vi "Save File Save Current.vi"(8 "Timer Seconds":dbl, 9 "Voltage":dbl, 10 "File Locations":T1, 11 "Current":dbl) -> (3 "Saving":bool)   [LabVIEW 2018, in "Save File.lvlib"]
uses:
  Save File.lvlib
  File Setup (Public)/Type Definition/Save File DOE File Path Control.ctl
  File Setup (Public)/Type Definition/Save File DOE Data Save Filepaths.ctl
  <vilib>/Utility/file.llb/Write To Spreadsheet File (string).vi
  <vilib>/Utility/file.llb/Write Delimited Spreadsheet (string).vi
  File Setup.lvlib
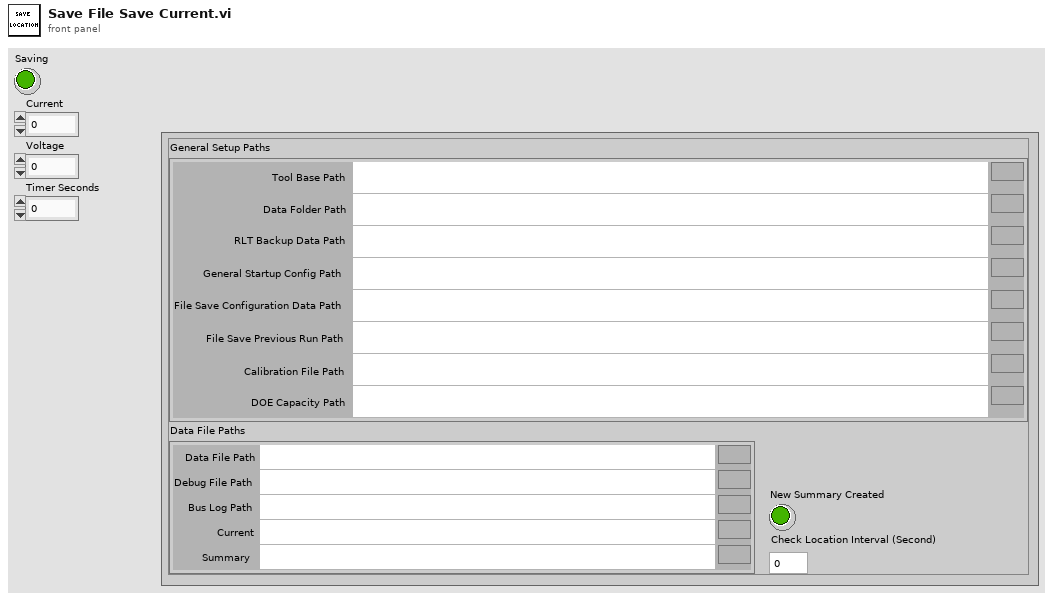
[diagram p1: front panel]
types:
  T1 = typedef "File Setup.lvlib/Save File DOE File Path Control.ctl" = cluster{"General Setup Paths":cluster{"Calibration File Path":path, "DOE Capacity Path":path, "Data Folder Path":path, "RLT Backup Data Path":path, "Tool Base Path":path, "General Startup Config Path":path, "File Save Previous Run Path":path, "File Save Configuration Data Path":path}, "Data File Paths":T2, "New Summary Created":bool, "Check Location Interval (Second)":i32}
  T2 = typedef "File Setup.lvlib/Save File DOE Data Save Filepaths.ctl" = cluster{"Data File Path":path, "Debug File Path":path, "Bus Log Path":path, "Current":path, "Summary":path}
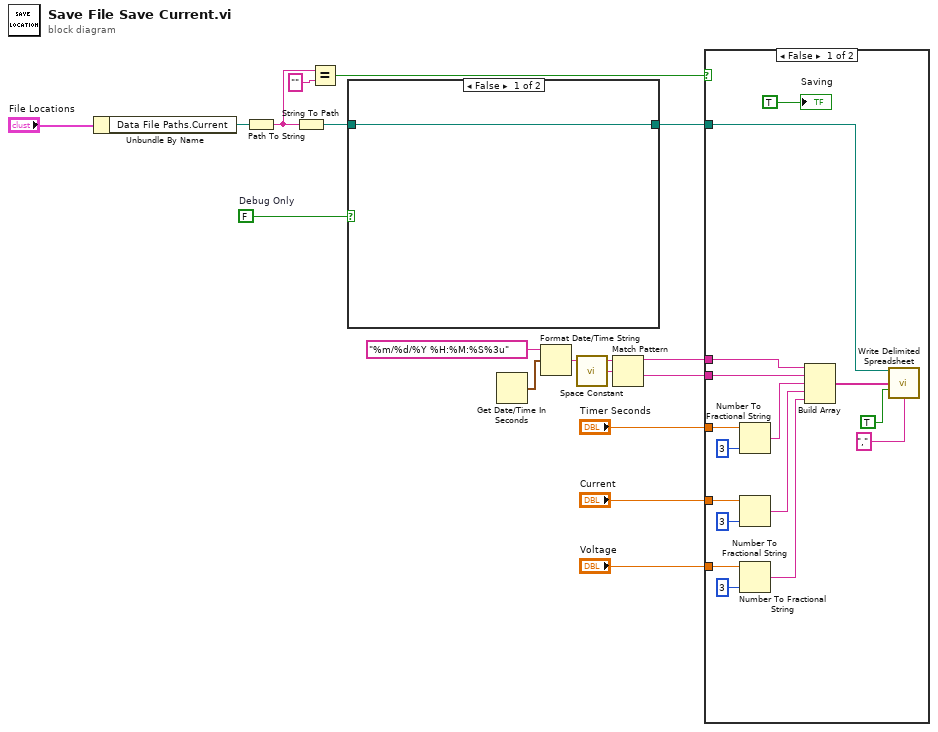
[diagram p0: block diagram]
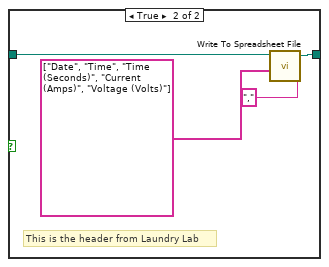
[diagram p2: hidden frame]
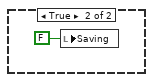
[diagram p3: hidden frame]
diagram:
  w4 = FALSE  # Debug Only
  n1 = Unbundle By Name("File Locations") -> ("Data File Paths.Current"=w6:path)
  n2 = Path To String(path=w6) -> (string=w5:string)
  n3 = String To Path(string=w5) -> (path=w3:path)
  n4 = Equal?(x=w5, y="") -> (x = y?=w16:bool)
  n5 = case shown="False" w4 {
    tunnel: w3 -> [w18 w21]
    tunnel: [w18 w20] -> w2
    frame False {
    }
    frame True {
      # "This is the header from Laundry Lab"
      n6 = call-poly <vilib>:"Write To Spreadsheet File.vi"("delimiter (\\t)"="," ("delimiter (\\t)"), "1D data"=string[] ["Date", "Time", "Time (Seconds)", "Current (Amps)", "Voltage (Volts)"] ("Current Header"), "file path (dialog if empty)"=w21) -> ("new file path (Not A Path if cancelled)"=w20:path)  [unwired: 5 in]
    }
  }
  n7 = Get Date/Time In Seconds() -> (seconds since 1Jan1904=w11:timestamp)
  n8 = Format Date/Time String(time format string (%c)="%m/%d/%Y %H:%M:%S%3u", seconds (now)=w11) -> (date/time string=w13:string)  [unwired: 1 in]
  n9 = call <vilib>:"Space Constant.vi"() -> ("String"=w14:string)
  n10 = Match Pattern(string=w13, regular expression=w14) -> (before substring=w9:string, after substring=w8:string)  [unwired: 1 in, 2 out]
  n11 = case shown="False" w16 {
    tunnel: "Current" -> [w38 _]
    tunnel: w2 -> [w37 _]
    tunnel: "Timer Seconds" -> [w36 _]
    tunnel: w9 -> [w35 _]
    tunnel: w8 -> [w34 _]
    tunnel: "Voltage" -> [w27 _]
    frame False {
      n12 = Number To Fractional String(number=w36, precision (6)=i16 3) -> (F-format string=w29:string)  [unwired: 2 in]
      n13 = Number To Fractional String(number=w38, precision (6)=i16 3) -> (F-format string=w31:string)  [unwired: 2 in]
      n14 = Number To Fractional String(number=w27, precision (6)=i16 3) -> (F-format string=w28:string)  [unwired: 2 in]
      n15 = Build Array(w35, w34, w29, w31, w28) -> (w23:string[])
      n16 = call-poly <vilib>:"Write Delimited Spreadsheet.vi"("file path (dialog if empty)"=w37, "1D data"=w23, "append to file? (new file:F)"=TRUE, "delimiter (\\t)"="," ("delimiter (\\t)")) -> ()  [unwired: 10 in, 2 out]
      "Saving" <- TRUE
    }
    frame True {
      n17 = local write "Saving"(FALSE ("Saving")) -> ()
    }
  }
